vi "CmdConsole.Read StdOut till Term Str or Timeout.vi"(7 "Match Line":bool, 8 "error in (no error)":errorcluster, 9 "Timeout(s)":dbl=5.0, 10 "TermStr":string, 11 "CmdConsole in":refnum<class "CmdConsole.lvclass">) -> (0 "error out":errorcluster, 1 "Lines":string[](array[string]), 2 "Data Present":bool, 3 "CmdConsole out":refnum<class "CmdConsole.lvclass">)   [LabVIEW 2024, in "CmdConsole.lvclass"]
uses:
  CmdConsole.lvclass
  CmdConsole.lvclass/CmdConsole.ctl
  <vilib>/Utility/error.llb/Trim Whitespace One-Sided.vi
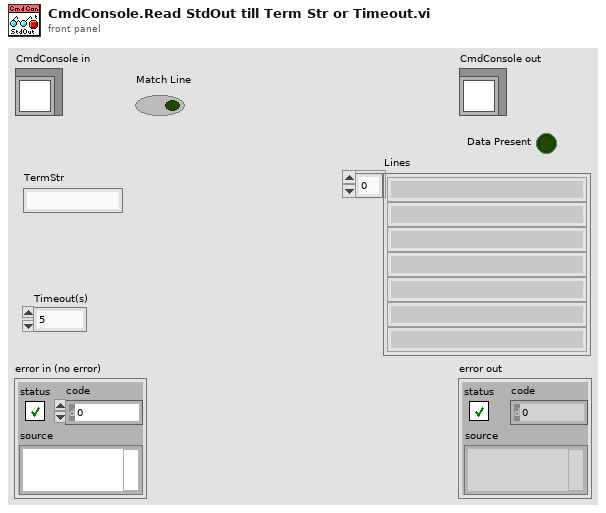
[diagram p1: front panel]
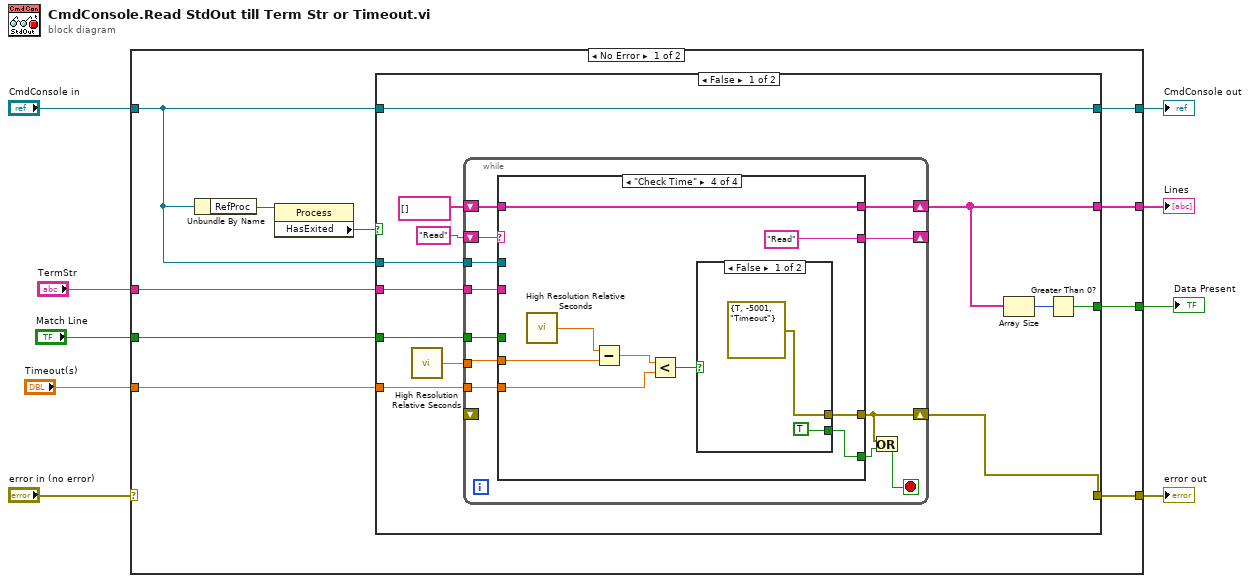
[diagram p0: block diagram]
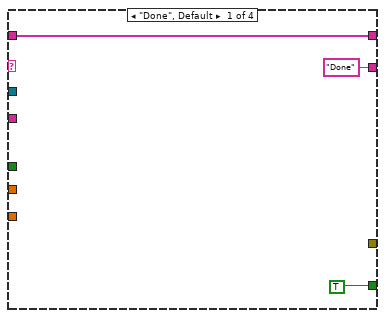
[diagram p2: hidden frame]
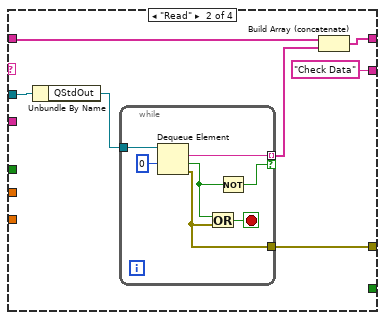
[diagram p3: hidden frame]
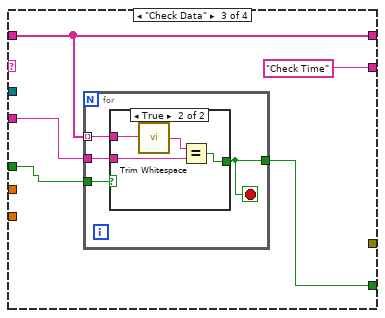
[diagram p4: hidden frame]
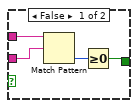
[diagram p5: hidden frame]
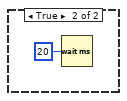
[diagram p6: hidden frame]
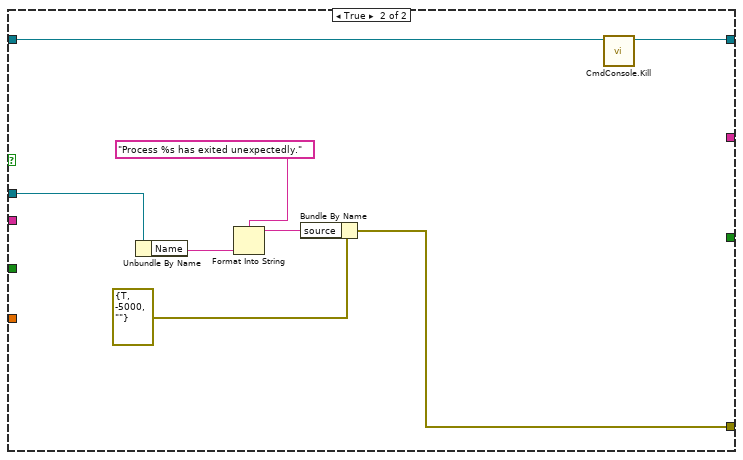
[diagram p7: hidden frame]
diagram:
  n1 = case shown="No Error" "error in (no error)" {
    selector: "error in (no error)" -> [_ w99]
    tunnel: [w16 w99] -> w8
    tunnel: [w13 w98] -> w6
    tunnel: "CmdConsole in" -> [w14 w98]
    tunnel: [w19 _] -> w5
    tunnel: [w18 _] -> w4
    tunnel: "Timeout(s)" -> [w12 _]
    tunnel: "TermStr" -> [w11 _]
    tunnel: "Match Line" -> [w10 _]
    frame No Error {
      n2 = Unbundle By Name(w14) -> ("RefProc"=w17:refnum<k24>)
      n3 = property class="Process"(reference=w17) -> ("HasExited"=w15:bool)  [unwired: 1 in, 2 out]
      n4 = case shown="False" w15 {
        tunnel: [w30 _] -> w19
        tunnel: [w21 _] -> w18
        tunnel: w14 -> [w29 w96]
        tunnel: [w27 w92] -> w16
        tunnel: w14 -> [w28 w91]
        tunnel: [w28 w90] -> w13
        tunnel: w12 -> [w23 _]
        tunnel: w11 -> [w22 _]
        tunnel: w10 -> [w20 _]
        frame False {
          n5 = call <vilib>:"High Resolution Relative Seconds.vi"() -> ("relative seconds"=w25:dbl)
          n6 = while {
            tunnel: w29 -> [w43]
            shift-right: [w40] -> w21
            shift-left: string[] [] -> [w41]
            tunnel: w25 -> [w36]
            shift-right: [w35] -> w27
            shift-left: _ -> [_]
            shift-right: [w39] -> _
            shift-left: "Read" -> [w42]
            tunnel: w23 -> [w38]
            tunnel: w22 -> [w37]
            tunnel: w20 -> [w32]
            stop <- w34 stop-if-true
            n7 = case shown="\"Check Time\"" w42 {
              tunnel: w43 -> [_ w52 _ _]
              tunnel: [_ w51 _ w78] -> w35
              tunnel: w41 -> [w46 w50 w65 w86]
              tunnel: [w46 w49 w65 w86] -> w40
              tunnel: ["Done" "Check Data" "Check Time" "Read"] -> w39
              tunnel: w38 -> [_ _ _ w82]
              tunnel: w37 -> [_ _ w62 _]
              tunnel: w36 -> [_ _ _ w85]
              tunnel: [TRUE _ w64 w80] -> w33
              tunnel: w32 -> [_ _ w61 _]
              frame "Done", Default {
              }
              frame "Read" {
                n8 = Unbundle By Name(w52) -> ("QStdOut"=w53:refnum<queue>)
                n9 = while {
                  tunnel: w53 -> [w60]
                  tunnel: [w58] -> w48 mode=indexing if=w57
                  tunnel: [w54] -> w51
                  stop <- w55 stop-if-true
                  n10 = Dequeue Element(queue=w60, timeout in ms (-1)=0) -> (element=w58:string, timed out?=w56:bool, error out=w54:errorcluster)  [unwired: 1 in, 1 out]
                  n11 = Or(x=w56, y=w54) -> (x .or. y?=w55:bool)
                  n12 = Not(x=w56) -> (.not. x?=w57:bool)
                }
                n13 = Build Array (concatenate)(w50, w48) -> (w49:string[])
              }
              frame "Check Data" {
                n14 = for {
                  tunnel: w65 -> [w69] mode=indexing
                  tunnel: [w68] -> w64
                  tunnel: w62 -> [w67]
                  tunnel: w61 -> [w66]
                  stop <- w68 stop-if-true
                  n15 = case shown="True" w66 {
                    tunnel: w69 -> [w73 w77]
                    tunnel: [w71 w75] -> w68
                    tunnel: w67 -> [w72 w74]
                    frame False {
                      n16 = Match Pattern(string=w73, regular expression=w72) -> (offset past match=w70:i32)  [unwired: 1 in, 3 out]
                      n17 = Greater Or Equal To 0?(x=w70) -> (x >= 0?=w71:bool)
                    }
                    frame True {
                      n18 = call <vilib>:"Trim Whitespace.vi"("string"=w77) -> ("trimmed string"=w76:string)  [unwired: 1 in]
                      n19 = Equal?(x=w76, y=w74) -> (x = y?=w75:bool)
                    }
                  }
                }
              }
              frame "Check Time" {
                n20 = call <vilib>:"High Resolution Relative Seconds.vi"() -> ("relative seconds"=w84:dbl)
                n21 = Subtract(x=w84, y=w85) -> (x-y=w83:dbl)
                n22 = Less?(x=w83, y=w82) -> (x < y?=w81:bool)
                n23 = case shown="False" w81 {
                  tunnel: [TRUE _] -> w80
                  tunnel: [errorcluster {"status"=TRUE, "code"=-5001, "source"="Timeout"} ("error constant") _] -> w78
                  frame False {
                  }
                  frame True {
                    n24 = Wait (ms)(milliseconds to wait=u32 20) -> ()  [unwired: 1 out]
                  }
                }
              }
            }
            n25 = Or(x=w35, y=w33) -> (x .or. y?=w34:bool)
          }
          n26 = Array Size(array=w21) -> (size(s)=w31:i32)
          n27 = Greater Than 0?(x=w31) -> (x > 0?=w30:bool)
        }
        frame True {
          n28 = Unbundle By Name(w96) -> ("Name"=w95:string)
          n29 = Format Into String(format string="Process %s has exited unexpectedly." ("source"), w95) -> (resulting string=w93:string)  [unwired: 2 in, 1 out]
          n30 = Bundle By Name(cluster=errorcluster {"status"=TRUE, "code"=-5000, "source"=""} ("error constant"), "source"=w93) -> (w92:errorcluster)
          n31 = call "CmdConsole.Kill.vi"("CmdConsole in"=w91) -> ("CmdConsole out"=w90:refnum<class "CmdConsole.lvclass">)  [unwired: 9 in, 1 out]
        }
      }
    }
    frame Error {
    }
  }
  "error out" <- w8
  "CmdConsole out" <- w6
  "Lines" <- w4
  "Data Present" <- w5
